vi "FGV.vi"(8 "error in":errorcluster, 9 "Use Simulated?":bool, 10 "Mode":T1, 11 "Database Record In":T2={"Door Open"=1.0, "Travel Time"=1.0, "Door Close"=1.0, "Inactivity Time"=1.0} {"Inactivity Time" format="%#_g Seconds"; "Door Close" format="%#_g Seconds"; "Travel Time" format="%#_g Seconds"; "Door Open" format="%#_g Seconds"}) -> (0 "error out":errorcluster, 3 "Database Record":T2={"Door Open"=1.0, "Travel Time"=1.0, "Door Close"=1.0, "Inactivity Time"=1.0} {"Inactivity Time" format="%#_g Seconds"; "Door Close" format="%#_g Seconds"; "Travel Time" format="%#_g Seconds"; "Door Open" format="%#_g Seconds"})   [LabVIEW 2020, in "Configuration Database.lvlib"]
doc: "FGV (Functional Global Variable) holding reference and internal data for the configuration database"
uses:
  Configuration Database.lvlib
  Controls/DB Record.ctl
  Controls/FGV Mode.ctl
  Controls/FGV Data.ctl
  Controls/Simulated Config Data.ctl
  Controls/RealDB Config Data.ctl
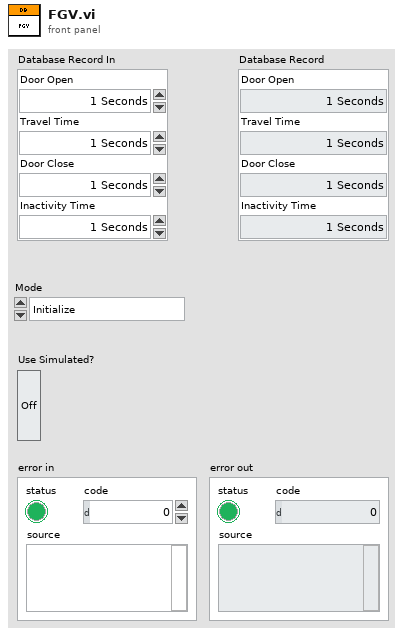
[diagram p1: front panel]
types:
  T1 = typedef "Configuration Database.lvlib/FGV Mode.ctl" = enum16{"Initialize", "Get", "Update", "Close"}
  T2 = typedef "Configuration Database.lvlib/DB Record.ctl" = cluster{"Door Open":dbl, "Travel Time":dbl, "Door Close":dbl, "Inactivity Time":dbl}
  T3 = typedef "Configuration Database.lvlib/FGV Data.ctl" = cluster{"Simulated Data":T4, "Real (Non-Simulated) Data":T5}
  T4 = typedef "Configuration Database.lvlib/Simulated Config Data.ctl" = cluster{"Config File Path":path}
  T5 = typedef "Configuration Database.lvlib/RealDB Config Data.ctl" = cluster{"Config File Path":path}
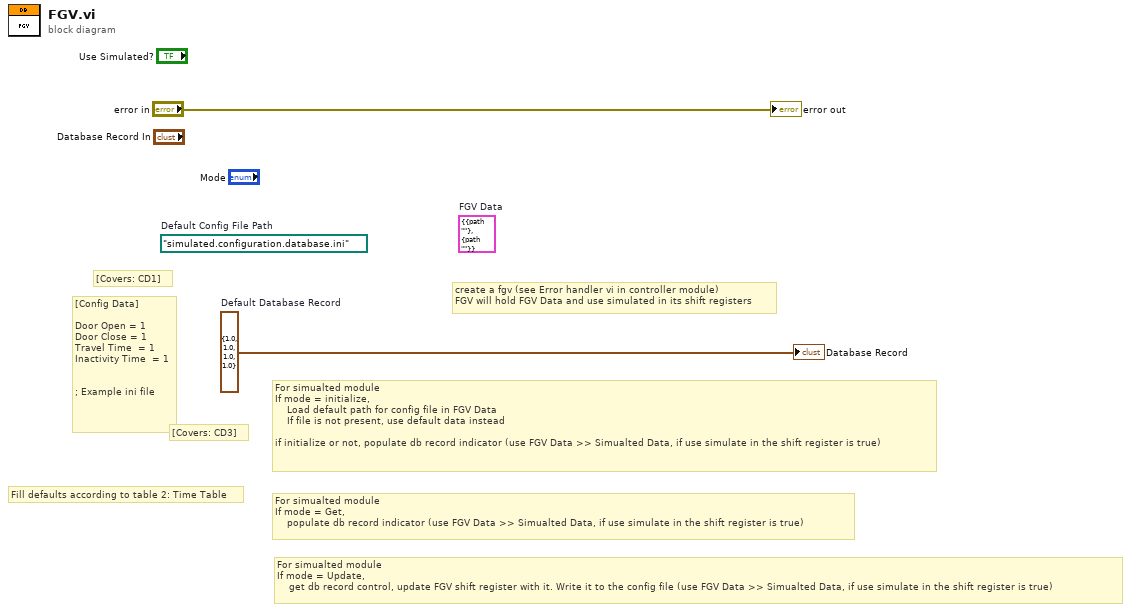
[diagram p0: block diagram]
diagram:
  w2 = T2 {"Door Open"=1.0, "Travel Time"=1.0, "Door Close"=1.0, "Inactivity Time"=1.0}  # Default Database Record
  (unwired) path "simulated.configuration.database.ini"  # Default Config File Path
  (unwired) T3 {"Simulated Data"={"Config File Path"=path ""}, "Real (Non-Simulated) Data"={"Config File Path"=path ""}}  # FGV Data
  # "Fill defaults according to table 2: Time Table"
  # "For simualted module\nIf mode = Update, \n    get db record control, update FGV shift register with it. Write it to the config file (use FGV Data >> Simualted Data, if use simulate in the shift register is true)"
  # "For simualted module\nIf mode = Get, \n    populate db record indicator (use FGV Data >> Simualted Data, if use simulate in the shift register is true)"
  # "[Covers: CD3]"
  # "[Config Data]\n\nDoor Open = 1\nDoor Close = 1\nTravel Time  = 1\nInactivity Time  = 1\n\n\n; Example ini file"
  # "[Covers: CD1]"
  # "For simualted module\nIf mode = initialize, \n    Load default path for config file in FGV Data\n    If file is not present, use default data instead\n\nif initialize or not, populate db record indicator (use FGV Data >> Simualted Data, if use simulate in the shift register is true)"
  # "create a fgv (see Error handler vi in controller module)\nFGV will hold FGV Data and use simulated in its shift registers"
  "error out" <- "error in"
  "Database Record" <- w2
